vi "Are All Channels Defined.vi"(10 "Channels":string[](array[string]), 11 "JSON RCT":refnum<class "JSON Routing Channel Template.lvclass">) -> (2 "All Defined?":bool, 3 "JSON RTC":refnum<class "JSON Routing Channel Template.lvclass">)   [LabVIEW 2020, in "Routing Templates.lvlib" / "JSON Routing Channel Template.lvclass"]
uses:
  JSON Routing Channel Template.lvclass
  C:/Users/mjacobso/Desktop/SCM/Routing-Faulting/Source/Routing and Faulting/Routing Templates/Routing Channel Templates/Abstract Routing Channel Template/Abstract Routing Channel Template.lvclass
  Abstract Routing Channel Template/Abstract Routing Channel Template.lvclass/Abstract Routing Channel Template.ctl
  Abstract Routing Channel Template/Read Channel Definition.vi
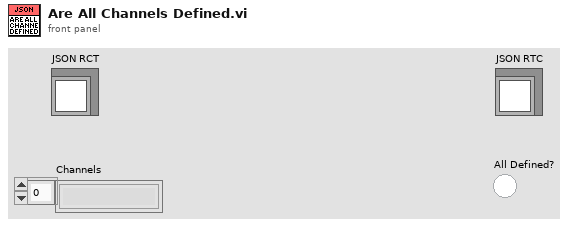
[diagram p1: front panel]
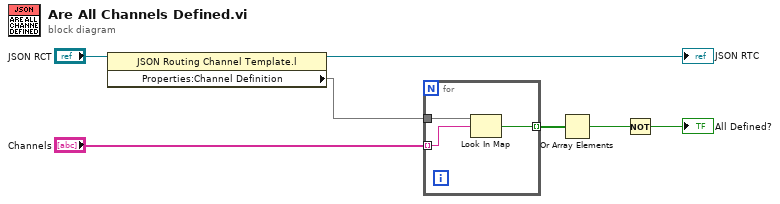
[diagram p0: block diagram]
diagram:
  n1 = property class="JSON Routing Channel Template.l"(reference="JSON RCT") -> (reference out=→"JSON RTC":refnum<class "JSON Routing Channel Template.lvclass">, "Properties:Channel Definition"=w4:map{string, string})  [unwired: 1 in, 1 out]
  n2 = for {
    tunnel: "Channels" -> [w9] mode=indexing
    tunnel: w4 -> [w10]
    tunnel: [w8] -> w3 mode=indexing
    n3 = Look In Map(map=w10, key=w9) -> (key not found?=w8:bool)  [unwired: 1 in, 1 out]
  }
  n4 = Or Array Elements(Boolean array=w3) -> (logical OR=w2:bool)
  n5 = Not(x=w2) -> (.not. x?=→"All Defined?":bool)
